vi "isInheritance.vi"(0 "reference":refnum<class "AbstractEdge.lvclass">, 5 "error in (no error)":errorcluster) -> (14 "reference out":refnum<class "AbstractEdge.lvclass">, 15 "isInheritance":bool, 16 "isCompAggregation":bool, 19 "error out":errorcluster)   [LabVIEW 2012, in "AbstractEdge.lvclass"]
doc: "Returns TRUE if Edge is a inheritance type"
uses:
  <resource>/Framework/Providers/Open_GDS/UML/AbstractEdge_class/AbstractEdge.lvclass
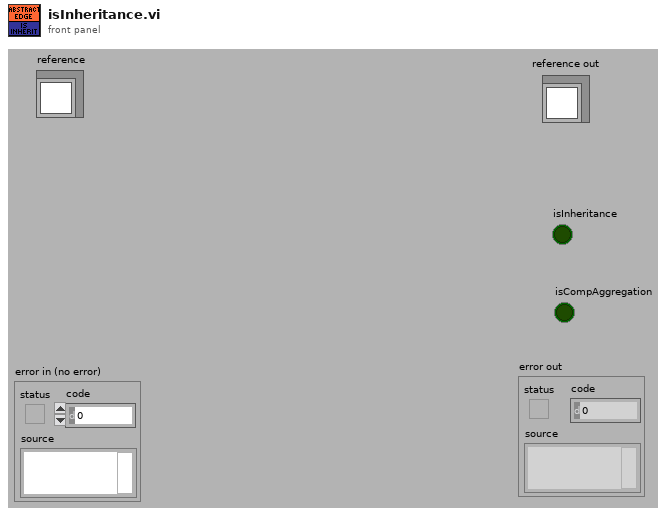
[diagram p1: front panel]
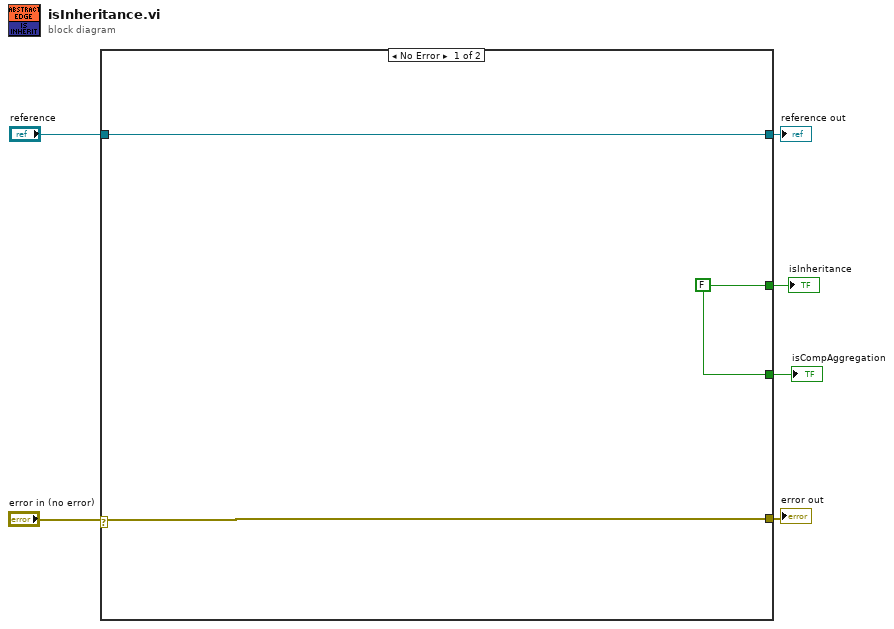
[diagram p0: block diagram]
diagram:
  n1 = case shown="No Error" "error in (no error)" {
    selector: "error in (no error)" -> [w8 w10]
    tunnel: "reference" -> [w9 w11]
    tunnel: [w8 w10] -> w5
    tunnel: [w9 w11] -> w4
    tunnel: [w7 _] -> w2
    tunnel: [w7 _] -> w1
    frame No Error {
      w7 = FALSE ("isInheritance")
    }
    frame Error {
    }
  }
  "reference out" <- w4
  "error out" <- w5
  "isInheritance" <- w2
  "isCompAggregation" <- w1
